vi "Values.vi"(11 "Result Row in":refnum<class "Result Row.lvclass">) -> (2 "Value":refnum<class "Type.lvclass">[](array[class]))   [LabVIEW 2020, in "Conditu2.lvlib" / "Result Row.lvclass"]
uses:
  Result Row.lvclass
  Columns/Type/Type.lvclass
  Result Row.lvclass/Result Row.ctl
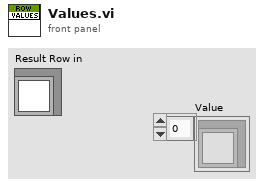
[diagram p1: front panel]
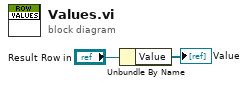
[diagram p0: block diagram]
diagram:
  n1 = Unbundle By Name("Result Row in") -> ("Value"=→"Value":refnum<class "Type.lvclass">[])
